vi "GUI.vi"(8 "error in":errorcluster, 9 "User Event Registration Refnum In":refnum<event-registration>) -> (0 "error out":errorcluster, 1 "User Event Registration Refnum Out":refnum<event-registration>)   [LabVIEW 2016]
uses:
  Generation/Oscillator/WaveformType.ctl
  DataEvent.ctl
  DataEvent/EventType.ctl
  GUI/ModulationControlEnum.ctl
  <vilib>/Analysis/3filter.llb/Filter Passband Type.ctl
  FGV/GetSetEnum.ctl
  FGV/ASIOData.ctl
  Generation/Filter/FilterInfo.ctl
  <vilib>/Analysis/NI_AALBase.lvlib
panel:
  in  "Settings Button":bool
  in  "order":i32(knob) scale=1.0..10.0
  in  "low cutoff freq":dbl(knob) scale=0.0..0.5 scale format="%#_6f"
  in  "high cutoff freq":dbl(knob) scale=0.0..0.5
  in  "filter type":T1
  in  "Feedback":bool
  in  "C:M ratio":i32(knob) scale=1.0..10.0 scale format="1 / %.0f"
  in  "Modulation control":T2
  in  "carrier frequency":dbl(knob)=10.0 scale=20.0..10000.0
  in  "modulator waveform":T3
  in  "Volume":dbl(slide)=1.0
  in  "modulation index":dbl(knob)=1.0 min=0.0 max=20.0 scale=0.0..20.0
  in  "modulation frequency":dbl(knob)=10.0 scale=1.0..10000.0
  in  "carrier waveform":T3
  out "Time signal":i32[](graph)
  out "Power spectrum":cluster{"f0":dbl, "df":dbl, "magnitude":dbl[]}(graph)
  in  "Play":bool
  in  "Exit":bool
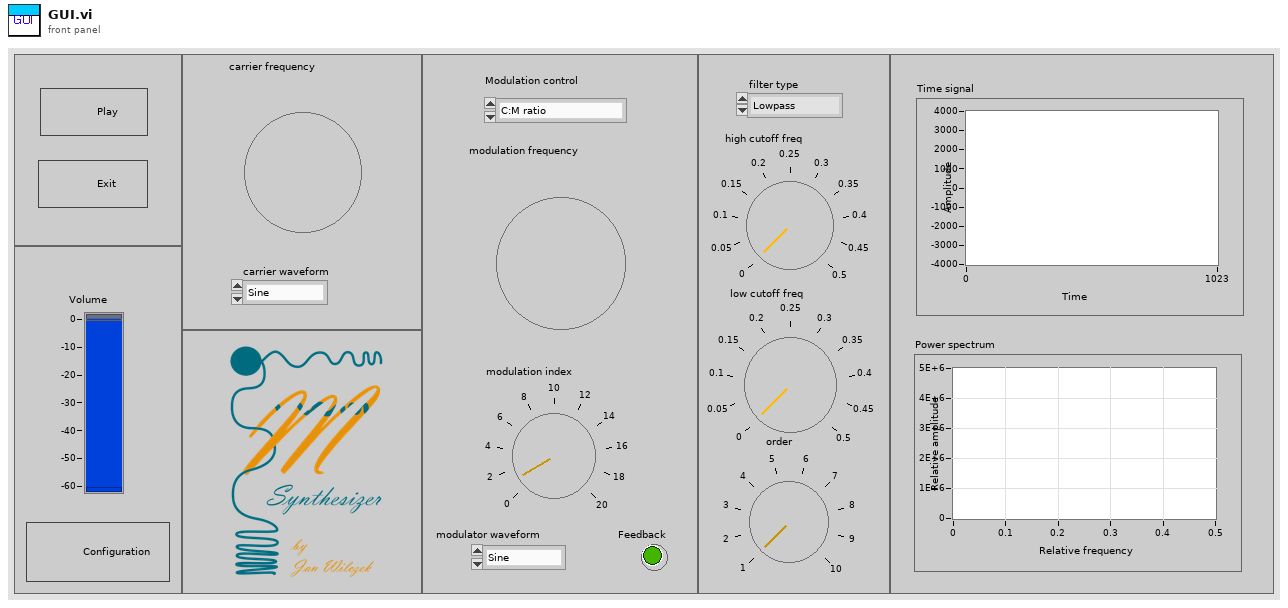
[diagram p1: front panel]
types:
  T1 = typedef "NI_AALBase.lvlib/Filter Passband Type.ctl" = enum32{"Lowpass", "Highpass", "Bandpass", "Bandstop"}
  T2 = typedef "ModulationControlEnum.ctl" = enum16{"C:M ratio", "Modulation frequency"}
  T3 = typedef "WaveformType.ctl" = enum16{"Sine", "Triangle", "Square", "Sawtooth"}
  T4 = typedef "GetSetEnum.ctl" = enum16{"Init", "Get", "Set"}
  T5 = typedef "FMInfo.ctl" = cluster{"buffer size":i32, "bits":i32, "CarrierInfo":cluster{"frequency":dbl, "amplitude":dbl, "sample rate":i32, "waveform type":T3}, "ModulatorInfo":cluster{"frequency":dbl, "amplitude":dbl, "sample rate":i32, "waveform type":T3}, "Feedback":bool}
  T6 = cluster{"frequency":dbl, "amplitude":dbl, "sample rate":i32, "waveform type":T3}
  T7 = typedef "FilterInfo.ctl" = cluster{"filter type":T1, "high cutoff freq: fh":dbl, "low cutoff freq: fl":dbl, "order":i32}
  T8 = typedef "ASIOData.ctl" = cluster{"Buffer Config":cluster{"# buffers":i32, "Buffer size":i32, "unit (ms)":enum16{"time (ms)", "Samples"}}, "Format (44kHz, 16Bit, stereo)":cluster{"Rate":i32, "Bits":i32, "Channels":u32}, "Play":bool, "Exit":bool}
  T9 = typedef "EventType.ctl" = enum16{"spectrum", "time", "exit"}
  T10 = cluster{"# buffers":i32, "Buffer size":i32, "unit (ms)":enum16{"time (ms)", "Samples"}}
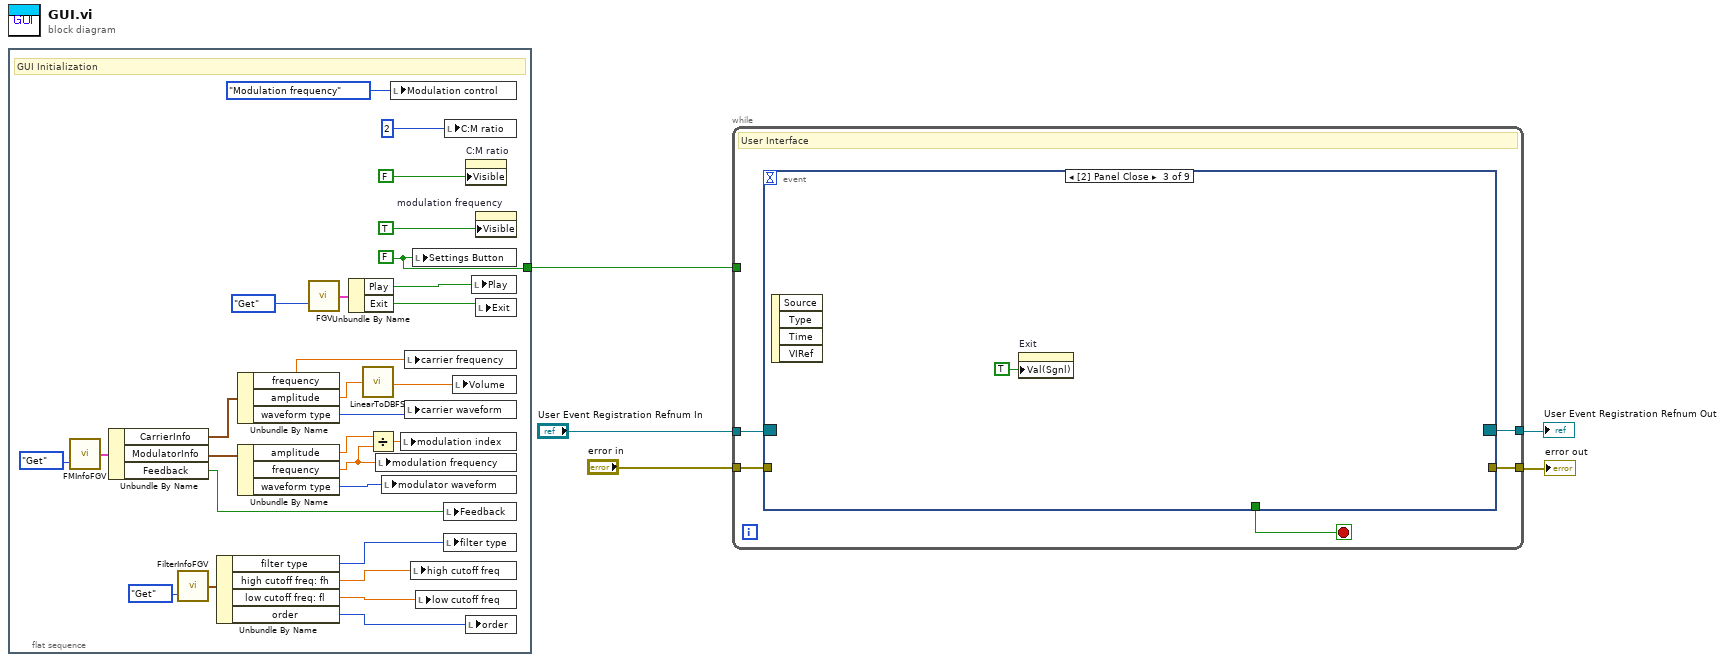
[diagram p0: block diagram]
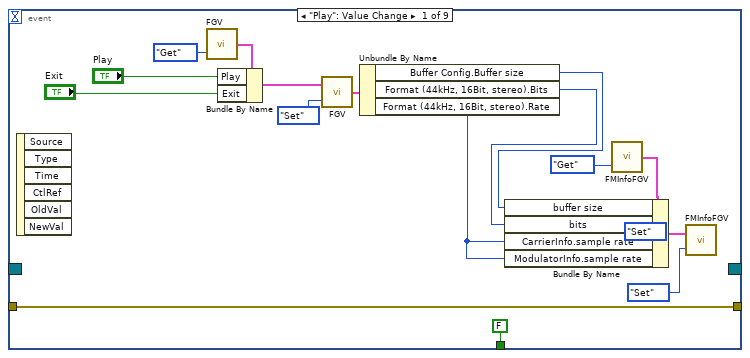
[diagram p2: hidden frame]
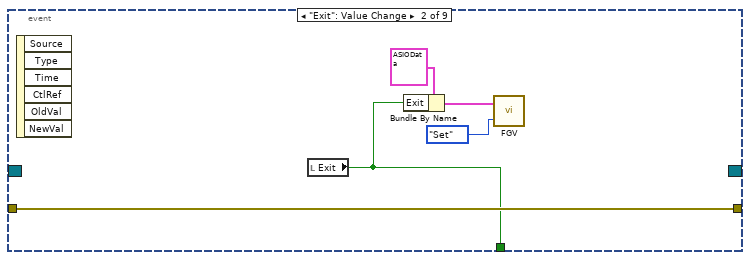
[diagram p3: hidden frame]
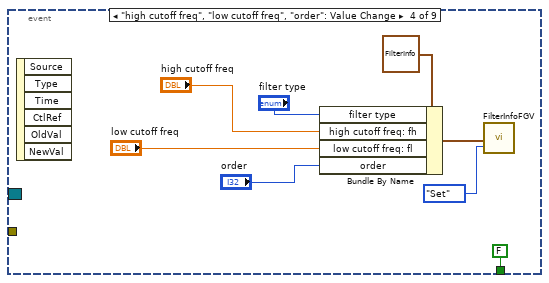
[diagram p4: hidden frame]
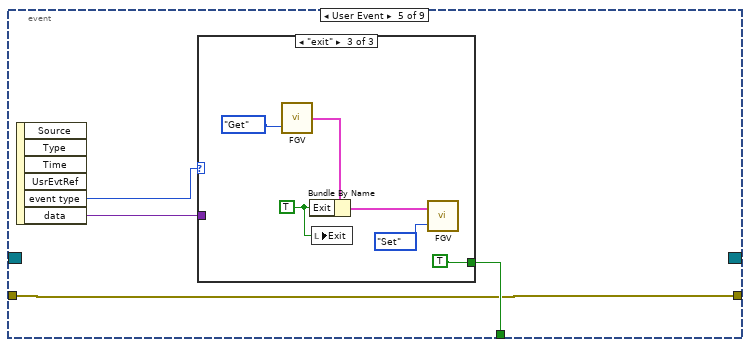
[diagram p5: hidden frame]
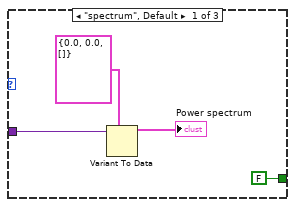
[diagram p6: hidden frame]
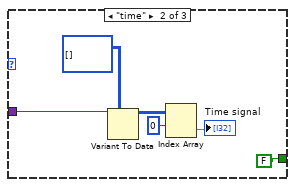
[diagram p7: hidden frame]
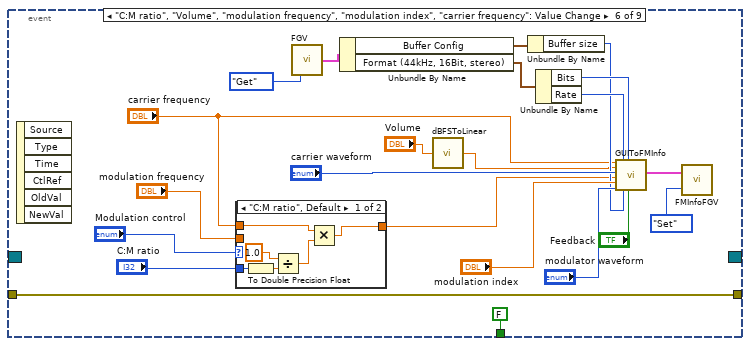
[diagram p8: hidden frame]
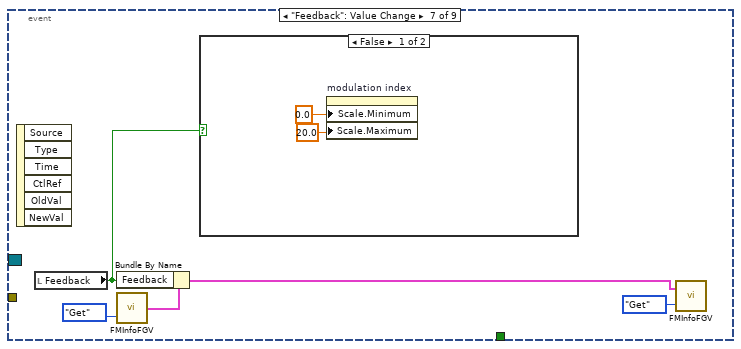
[diagram p10: hidden frame]
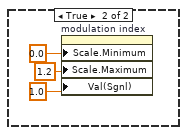
[diagram p11: hidden frame]
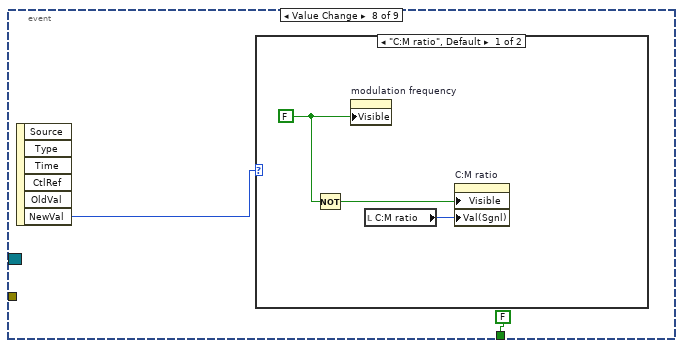
[diagram p12: hidden frame]
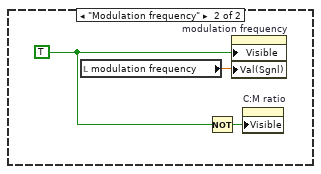
[diagram p13: hidden frame]
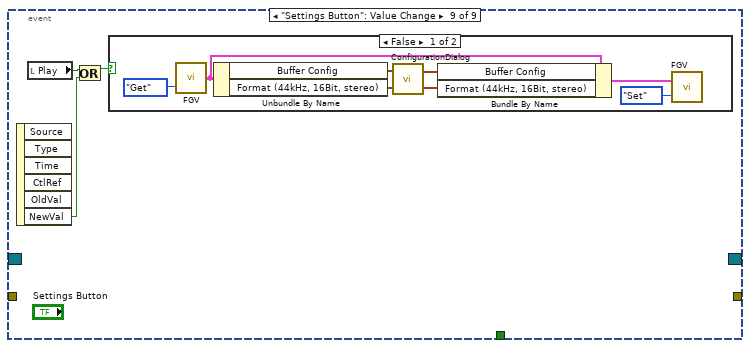
[diagram p14: hidden frame]
diagram:
  n1 = flat-sequence {
    tunnel: [w9] -> w1
    frame #0 {
      w9 = FALSE ("Settings Button")
      # "GUI Initialization"
      n2 = call "FMInfoFGV.vi"("GetSetEnum"=GetSetEnum."Get") -> ("FMInfoOut"=w22:T5)  [unwired: 1 in]
      n3 = Unbundle By Name(w22) -> ("CarrierInfo"=w16:T6, "ModulatorInfo"=w15:T6, "Feedback"=w17:bool)
      n4 = call "FilterInfoFGV.vi"("GetSet enum"=GetSetEnum."Get") -> ("FilterInfo out"=w28:T7)  [unwired: 1 in]
      n5 = Unbundle By Name(w28) -> ("filter type"=w27:T1, "high cutoff freq: fh"=w26:dbl, "low cutoff freq: fl"=w25:dbl, "order"=w24:i32)
      n6 = Unbundle By Name(w16) -> ("frequency"=w14:dbl, "amplitude"=w6:dbl, "waveform type"=w13:T3)
      n7 = Unbundle By Name(w15) -> ("amplitude"=w8:dbl, "frequency"=w7:dbl, "waveform type"=w12:T3)
      n8 = call "FGV.vi"("GetSetEnum"=GetSetEnum."Get") -> ("ASIODataOut"=w20:T8)  [unwired: 1 in]
      n9 = Unbundle By Name(w20) -> ("Play"=w18:bool, "Exit"=w19:bool)
      n10 = call "LinearToDBFS.vi"("Linear"=w6) -> ("dBFS"=w11:dbl)
      n11 = Divide(x=w8, y=w7) -> (x/y=w10:dbl)
      n12 = local write "modulation frequency"(w7) -> ()
      n13 = local write "modulator waveform"(w12) -> ()
      n14 = local write "Modulation control"(ModulationControlEnum."Modulation frequency" ("Modulation control")) -> ()
      n15 = local write "modulation index"(w10) -> ()
      n16 = local write "carrier frequency"(w14) -> ()
      n17 = local write "carrier waveform"(w13) -> ()
      n18 = local write "high cutoff freq"(w26) -> ()
      n19 = local write "Settings Button"(w9) -> ()
      n20 = local write "low cutoff freq"(w25) -> ()
      n21 = local write "Feedback"(w17) -> ()
      n22 = local write "filter type"(w27) -> ()
      n23 = local write "C:M ratio"(2 ("C:M ratio")) -> ()
      n24 = local write "Volume"(w11) -> ()
      n25 = property on="C:M ratio" class="Knob (strict)"("Visible"=FALSE) -> ()  [unwired: 2 in, 2 out]
      n26 = local write "order"(w24) -> ()
      n27 = local write "Play"(w18) -> ()
      n28 = property on="modulation frequency" class="Knob (strict)"("Visible"=TRUE) -> ()  [unwired: 2 in, 2 out]
      n29 = local write "Exit"(w19) -> ()
    }
  }
  n30 = while {
    tunnel: "User Event Registration Refnum In" -> [w37]
    tunnel: [w36] -> w2
    tunnel: "error in" -> [w35]
    tunnel: [w34] -> w5
    tunnel: w1 -> [_]
    stop <- w38 stop-if-true
    # "User Interface"
    n31 = event shown="[2] Panel Close" {
      selector: w37 -> [_ _ _ _ _ _ _ _ _]
      dyn-events: [_ _ _ _ _ _ _ _ _] -> w36
      timeout: _ -> [_ _ _ _ _ _ _ _ _]
      tunnel: [FALSE ("Exit") w55 _ FALSE ("Exit") w70 FALSE ("Exit") _ FALSE ("Exit") _] -> w38
      tunnel: w35 -> [w51 w59 _ _ w69 w104 _ _ _]
      tunnel: [w51 w59 _ _ w69 w104 _ _ _] -> w34
      event "Play": Value Change {
        (unwired) GetSetEnum."Set" ("GetSetEnum")
        n32 = event-data() -> ()  [unwired: 1 in, 6 out]
        n33 = call "FGV.vi"("GetSetEnum"=GetSetEnum."Get") -> ("ASIODataOut"=w48:T8)  [unwired: 1 in]
        n34 = Bundle By Name(cluster=w48, "Play"="Play", "Exit"="Exit") -> (w47:T8)
        n35 = call "FGV.vi"("GetSetEnum"=GetSetEnum."Set", "ASIODataIn"=w47) -> ("ASIODataOut"=w45:T8)
        n36 = Unbundle By Name(w45) -> ("Buffer Config.Buffer size"=w43:i32, "Format (44kHz, 16Bit, stereo).Bits"=w42:i32, "Format (44kHz, 16Bit, stereo).Rate"=w41:i32)
        n37 = call "FMInfoFGV.vi"("GetSetEnum"=GetSetEnum."Get") -> ("FMInfoOut"=w44:T5)  [unwired: 1 in]
        n38 = Bundle By Name(cluster=w44, "buffer size"=w43, "bits"=w42, "CarrierInfo.sample rate"=w41, "ModulatorInfo.sample rate"=w41) -> (w40:T5)
        n39 = call "FMInfoFGV.vi"("GetSetEnum"=GetSetEnum."Set", "FMInfoIn"=w40) -> ()  [unwired: 1 out]
      }
      event "Exit": Value Change {
        n40 = event-data() -> ()  [unwired: 1 in, 6 out]
        n41 = local read "Exit"() -> (w55:bool)
        n42 = Bundle By Name(cluster=T8 {"Buffer Config"={"# buffers"=4, "Buffer size"=2048, "unit (ms)"=enum."Samples"}, "Format (44kHz, 16Bit, stereo)"={"Rate"=44100, "Bits"=16, "Channels"=2}, "Play"=FALSE, "Exit"=FALSE} ("ASIODataIn"), "Exit"=w55) -> (w57:T8)
        n43 = call "FGV.vi"("GetSetEnum"=GetSetEnum."Set", "ASIODataIn"=w57) -> ()  [unwired: 1 out]
      }
      event Panel Close {
        n44 = event-data() -> ()  [unwired: 1 in, 4 out]
        n45 = property on="Exit" class="Bool (strict)"("Val(Sgnl)"=TRUE ("Value (Signaling)")) -> ()  [unwired: 2 in, 2 out]
      }
      event "high cutoff freq", "low cutoff freq", "order": Value Change {
        n46 = event-data() -> ()  [unwired: 1 in, 6 out]
        n47 = Bundle By Name(cluster=T7 {"filter type"=enum."Lowpass", "high cutoff freq: fh"=0.45000000000000007, "low cutoff freq: fl"=0.12500000000000006, "order"=2} ("FilterInfo"), "filter type"="filter type", "high cutoff freq: fh"="high cutoff freq", "low cutoff freq: fl"="low cutoff freq", "order"="order") -> (w63:T7)
        n48 = call "FilterInfoFGV.vi"("GetSet enum"=GetSetEnum."Set", "FilterInfo in"=w63) -> ()  [unwired: 1 out]
      }
      event User Event {
        n49 = event-data() -> ("event type"=w72:T9, "data"=w71:variant)  [unwired: 1 in, 4 out]
        n50 = case shown="\"exit\"" w72 {
          tunnel: w71 -> [w76 w82 _]
          tunnel: [FALSE ("Exit") FALSE ("Exit") TRUE ("Exit")] -> w70
          frame "spectrum", Default {
            n51 = Variant To Data(type=cluster{"f0":dbl, "df":dbl, "magnitude":dbl[]} {"f0"=0.0, "df"=0.0, "magnitude"=[]} ("Power Spectrum / PSD"), Variant=w76) -> (data=→"Power spectrum":cluster{"f0":dbl, "df":dbl, "magnitude":dbl[]})  [unwired: 1 in, 1 out]
          }
          frame "time" {
            n52 = Variant To Data(type=i32[][] [] ("signal for ASIO"), Variant=w82) -> (data=w79:i32[][])  [unwired: 1 in, 1 out]
            n53 = Index Array(array=w79, index (row)=0) -> (element=→"Time signal":i32[])  [unwired: 1 in]
          }
          frame "exit" {
            w83 = TRUE ("Exit")
            n54 = call "FGV.vi"("GetSetEnum"=GetSetEnum."Get") -> ("ASIODataOut"=w84:T8)  [unwired: 1 in]
            n55 = Bundle By Name(cluster=w84, "Exit"=w83) -> (w86:T8)
            n56 = local write "Exit"(w83) -> ()
            n57 = call "FGV.vi"("GetSetEnum"=GetSetEnum."Set", "ASIODataIn"=w86) -> ()  [unwired: 1 out]
          }
        }
      }
      event "C:M ratio", "Volume", "modulation frequency", "modulation index", "carrier frequency": Value Change {
        n58 = event-data() -> ()  [unwired: 1 in, 6 out]
        n59 = case shown="\"C:M ratio\", Default" "Modulation control" {
          tunnel: "modulation frequency" -> [_ w117]
          tunnel: [w113 w117] -> w93
          tunnel: "carrier frequency" -> [w112 _]
          tunnel: "C:M ratio" -> [w115 _]
          frame "C:M ratio", Default {
            n60 = To Double Precision Float(number=w115) -> (double precision float=w114:dbl)
            n61 = Divide(x=1.0, y=w114) -> (x/y=w111:dbl)
            n62 = Multiply(x=w112, y=w111) -> (x*y=w113:dbl)
          }
          frame "Modulation frequency" {
          }
        }
        n63 = call "FGV.vi"("GetSetEnum"=GetSetEnum."Get") -> ("ASIODataOut"=w103:T8)  [unwired: 1 in]
        n64 = Unbundle By Name(w103) -> ("Buffer Config"=w102:T10, "Format (44kHz, 16Bit, stereo)"=w101:cluster{"Rate":i32, "Bits":i32, "Channels":u32})
        n65 = call "dBFSToLinear.vi"("dBFS"="Volume") -> ("Linear"=w97:dbl)
        n66 = Unbundle By Name(w102) -> ("Buffer size"=w98:i32)
        n67 = Unbundle By Name(w101) -> ("Bits"=w100:i32, "Rate"=w99:i32)
        n68 = call "GUIToFMInfo.vi"("carrier frequency"="carrier frequency", "amplitude"=w97, "carrier waveform"="carrier waveform", "modulation frequency"=w93, "modulation index"="modulation index", "modulator waveform"="modulator waveform", "sample rate"=w99, "buffer size"=w98, "bits"=w100, "Feedback"="Feedback") -> ("FMInfo"=w90:T5)  [unwired: 9 in]
        n69 = call "FMInfoFGV.vi"("GetSetEnum"=GetSetEnum."Set", "FMInfoIn"=w90) -> ()  [unwired: 1 out]
      }
      event "Feedback": Value Change {
        n70 = event-data() -> ()  [unwired: 1 in, 6 out]
        n71 = local read "Feedback"() -> (w118:bool)
        n72 = call "FMInfoFGV.vi"("GetSetEnum"=GetSetEnum."Get") -> ("FMInfoOut"=w120:T5)  [unwired: 1 in]
        n73 = Bundle By Name(cluster=w120, "Feedback"=w118) -> (w119:T5)
        n74 = case shown="False" w118 {
          frame False {
            n75 = property on="modulation index" class="Knob (strict)"("Scale.Minimum"=0.0 ("Data Entry Limits:Minimum"), "Scale.Maximum"=20.0 ("Data Entry Limits:Maximum")) -> ()  [unwired: 2 in, 2 out]
          }
          frame True {
            n76 = property on="modulation index" class="Knob (strict)"("Scale.Minimum"=0.0 ("Data Entry Limits:Minimum"), "Scale.Maximum"=1.2 ("Data Entry Limits:Maximum"), "Val(Sgnl)"=1.0 ("Value (Signaling)")) -> ()  [unwired: 2 in, 2 out]
          }
        }
        n77 = call "FMInfoFGV.vi"("GetSetEnum"=GetSetEnum."Get", "FMInfoIn"=w119) -> ()  [unwired: 1 out]
      }
      event Value Change {
        n78 = event-data() -> ("NewVal"=w129:T2)  [unwired: 1 in, 5 out]
        n79 = case shown="\"C:M ratio\", Default" w129 {
          frame "C:M ratio", Default {
            w132 = FALSE ("Visible")
            n80 = Not(x=w132) -> (.not. x?=w131:bool)
            n81 = property on="modulation frequency" class="Knob (strict)"("Visible"=w132) -> ()  [unwired: 2 in, 2 out]
            n82 = local read "C:M ratio"() -> (w130:i32)
            n83 = property on="C:M ratio" class="Knob (strict)"("Visible"=w131, "Val(Sgnl)"=w130) -> ()  [unwired: 2 in, 2 out]
          }
          frame "Modulation frequency" {
            w135 = TRUE ("Visible")
            n84 = local read "modulation frequency"() -> (w133:dbl)
            n85 = Not(x=w135) -> (.not. x?=w134:bool)
            n86 = property on="modulation frequency" class="Knob (strict)"("Visible"=w135, "Val(Sgnl)"=w133) -> ()  [unwired: 2 in, 2 out]
            n87 = property on="C:M ratio" class="Knob (strict)"("Visible"=w134) -> ()  [unwired: 2 in, 2 out]
          }
        }
      }
      event "Settings Button": Value Change {
        n88 = event-data() -> ("NewVal"=w137:bool)  [unwired: 1 in, 5 out]
        n89 = local read "Play"() -> (w138:bool)
        n90 = Or(x=w138, y=w137) -> (x .or. y?=w136:bool)
        n91 = case shown="False" w136 {
          frame False {
            n92 = call "FGV.vi"("GetSetEnum"=GetSetEnum."Get") -> ("ASIODataOut"=w142:T8)  [unwired: 1 in]
            n93 = Unbundle By Name(w142) -> ("Buffer Config"=w145:T10, "Format (44kHz, 16Bit, stereo)"=w144:cluster{"Rate":i32, "Bits":i32, "Channels":u32})
            n94 = call "ConfigurationDialog.vi"("Format In"=w144, "Buffer Config In"=w145) -> ("Format Out"=w140:cluster{"Rate":i32, "Bits":i32, "Channels":u32}, "Buffer Config Out"=w141:T10)
            n95 = Bundle By Name(cluster=w142, "Buffer Config"=w141, "Format (44kHz, 16Bit, stereo)"=w140) -> (w139:T8)
            n96 = call "FGV.vi"("GetSetEnum"=GetSetEnum."Set", "ASIODataIn"=w139) -> ()  [unwired: 1 out]
          }
          frame True {
          }
        }
      }
    }
  }
  "error out" <- w5
  "User Event Registration Refnum Out" <- w2
